vi "GoTarget.vi"(6 "Enable ND":bool, 8 "max speed":dbl=0.35, 9 "Distance":dbl=0.02, 10 "SubGoal":dbl[](array[numeric]), 11 "Odometry Data":dbl[](array[numeric])) -> (0 "Target Distance":dbl, 1 "Head CMD":dbl, 2 "VY":dbl, 3 "VX":dbl)   [LabVIEW 2018]
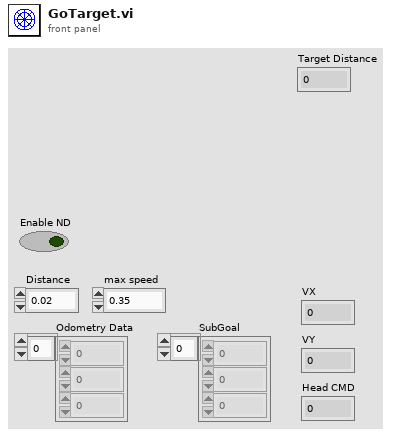
[diagram p1: front panel]
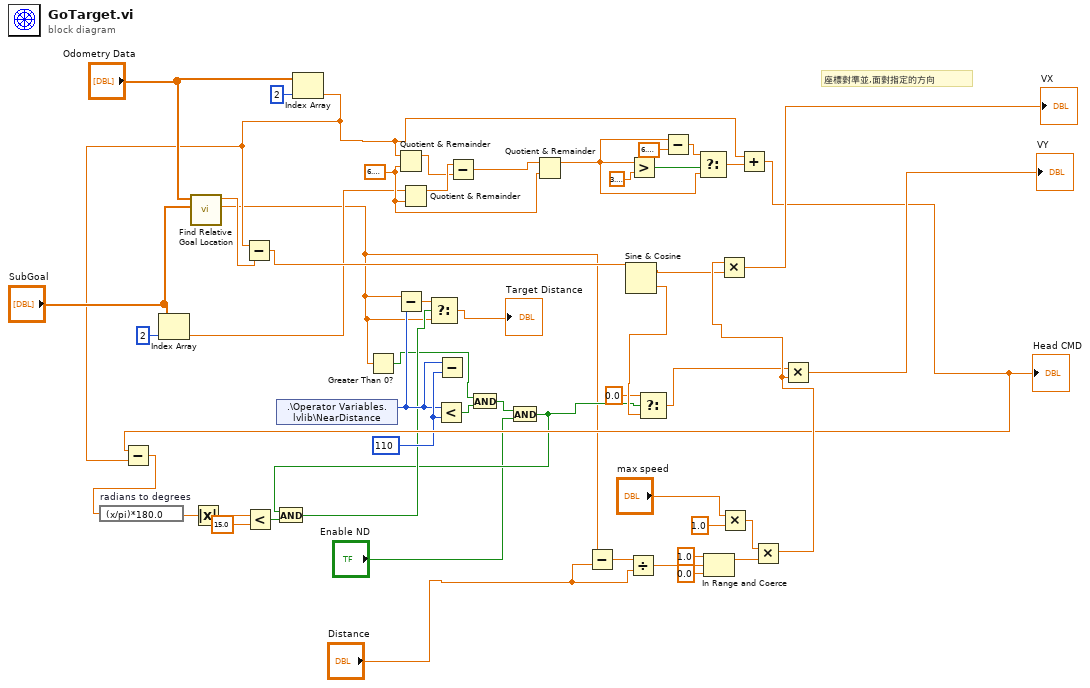
[diagram p0: block diagram]
diagram:
  w12 = 110 ("y")
  w30 = 6.283185307179586
  # "座標對準並,面對指定的方向"
  n1 = Index Array(array="SubGoal", index=2) -> (element=w23:dbl)
  n2 = call "Find Relative Goal Location.vi"("Goal Position"="SubGoal", "Current Position"="Odometry Data") -> ("Target Distance"=w5:dbl, "Target Heading"=w48:dbl)  [unwired: 8 in]
  n3 = shared-variable ".\\Operator Variables.lvlib\\NearDistance"() -> (w10:i32)  [unwired: 1 in, 1 out]
  n4 = Index Array(array="Odometry Data", index=2) -> (element=w15:dbl)
  n5 = Subtract(x=w15, y=w48) -> (x-y=w47:dbl)
  n6 = Greater Than 0?(x=w5) -> (x > 0?=w3:bool)
  n7 = Quotient & Remainder(x=w15, y=w30) -> (x-y*floor(x/y)=w32:dbl)  [unwired: 1 out]
  n8 = Subtract(x=w5, y=w10) -> (x-y=w11:dbl)
  n9 = Quotient & Remainder(x=w23, y=w30) -> (x-y*floor(x/y)=w33:dbl)  [unwired: 1 out]
  n10 = Less?(x=w10, y=w12) -> (x < y?=w4:bool)
  n11 = Subtract(x=w10, y=w12) -> ()  [unwired: 1 out]
  n12 = Subtract(x=w33, y=w32) -> (x-y=w31:dbl)
  n13 = And(x=w3, y=w4) -> (x .and. y?=w2:bool)
  n14 = And(x=w2, y="Enable ND") -> (x .and. y?=w7:bool)
  n15 = Quotient & Remainder(x=w31, y=w30) -> (x-y*floor(x/y)=w25:dbl)  [unwired: 1 out]
  n16 = Subtract(x=w5, y="Distance") -> (x-y=w42:dbl)
  n17 = Sine & Cosine(0:w47) -> (1:w22:dbl, 2:w21:dbl)
  n18 = Divide(x=w42, y="Distance") -> (x/y=w43:dbl)
  n19 = Greater?(x=w25, y=3.141592653589793) -> (0:w28:bool)
  n20 = Select(t=0.0, s=w7, f=w21) -> (s? t:f=w20:dbl)
  n21 = Subtract(x=w25, y=6.283185307179586) -> (x-y=w26:dbl)
  n22 = Select(t=w26, s=w28, f=w25) -> (s? t:f=w24:dbl)
  n23 = In Range and Coerce(upper limit=1.0, x=w43, lower limit=0.0) -> (coerced(x)=w45:dbl)  [unwired: 1 out]
  n24 = Multiply(x="max speed", y=1.0) -> (x*y=w51:dbl)
  n25 = Add(x=w15, y=w24) -> (x+y=w14:dbl)
  "Head CMD" <- w14
  n26 = Subtract(x=w14, y=w15) -> (x-y=w17:dbl)
  n27 = expression code="(x/pi)*180.0" "radians to degrees"(w17) -> (w16:dbl)
  n28 = Absolute Value(x=w16) -> (abs(x)=w18:dbl)
  n29 = Less?(x=w18, y=15.0) -> (x < y?=w13:bool)
  n30 = And(x=w7, y=w13) -> (x .and. y?=w9:bool)
  n31 = Select(t=w11, s=w9, f=w5) -> (s? t:f=→"Target Distance":dbl)
  n32 = Multiply(x=w51, y=w45) -> (x*y=w46:dbl)
  n33 = Multiply(x=w46, y=w22) -> (x*y=→"VX":dbl)
  n34 = Multiply(x=w20, y=w46) -> (x*y=→"VY":dbl)
